vi "F11xx_FileMerger_V2.vi"() -> ()   [LabVIEW 2018]
uses:
  <vilib>/Utility/file.llb/Read From Spreadsheet File (string).vi
  <vilib>/Utility/file.llb/Write To Spreadsheet File (string).vi
panel:
  in  "Header Row":i32=42
  out "Array 4":i32[](array[numeric])=[37, 36, 36, 36, 36, 36, 36, 36, 36, 36, 36, 36, 36, 36, 36, 36, 36, 36, 36, 36, 36, 36]
  out "Array 3":bool[](array[boolean])
  out "Array 2":string[](array[string])=["10", "11", "12", "13", "14", "15", "16", "17", "18", "19", "1", "20", "21", "22", "2", "3", "4", "5", "6", "7", "8", "9"]
  out "Boolean":bool
  in  "Write to File":bool
  in  "Folder":path=path "\\\\Corpmxl0251xct\\c/IdtATE/Results/Loadbrd _r2_firstlook_F1150_080811/EvKit Plunge"
  in  "Target File":path=path "\\\\Corpmxl0251xct\\c/IdtATE/Results/Loadbrd _r2_firstlook_F1150_080811/EvKit Plunge/Loadbrd _r2_firstlook_F1150_080811_SN_1Thru22.csv"
  in  "offset (0) 2":i32=40
  in  "offset (0)":i32=11
  out "Array":string[](array[string])=["9", "9", "9", "9", "9", "9", "9", "9", "9", "9", "9", "9", "9", "9", "9", "9", "9", "9", "9", "9", "9", "9", "9", "9", "9", "9", "9", "9", "9", "9", "9", "9", "9", "9", "9", "9"]
  out "element":i32=36
  out "filenames":string[](array[string])=["Loadbrd _r2_firstlook_F1150_080811_SN_1-10_151403.csv", "Loadbrd _r2_firstlook_F1150_080811_SN_1-11_152349.csv", "Loadbrd _r2_firstlook_F1150_080811_SN_1-12_153322.csv", "Loadbrd _r2_firstlook_F1150_080811_SN_1-13_154231.csv", "Loadbrd _r2_firstlook_F1150_080811_SN_1-14_155132.csv", "Loadbrd _r2_firstlook_F1150_080811_SN_1-15_160102.csv", "Loadbrd _r2_firstlook_F1150_080811_SN_1-16_161750.csv", "Loadbrd _r2_firstlook_F1150_080811_SN_1-17_162638.csv", "Loadbrd _r2_firstlook_F1150_080811_SN_1-18_163501.csv", "Loadbrd _r2_firstlook_F1150_080811_SN_1-19_164508.csv", "Loadbrd _r2_firstlook_F1150_080811_SN_1-1_134125.csv", "Loadbrd _r2_firstlook_F1150_080811_SN_1-20_165401.csv", "Loadbrd _r2_firstlook_F1150_080811_SN_1-21_170335.csv", "Loadbrd _r2_firstlook_F1150_080811_SN_1-22_171202.csv", "Loadbrd _r2_firstlook_F1150_080811_SN_1-2_135257.csv", "Loadbrd _r2_firstlook_F1150_080811_SN_1-3_140438.csv", "Loadbrd _r2_firstlook_F1150_080811_SN_1-4_141457.csv", "Loadbrd _r2_firstlook_F1150_080811_SN_1-5_142448.csv", "Loadbrd _r2_firstlook_F1150_080811_SN_1-6_143320.csv", "Loadbrd _r2_firstlook_F1150_080811_SN_1-7_144223.csv", "Loadbrd _r2_firstlook_F1150_080811_SN_1-8_145159.csv", "Loadbrd _r2_firstlook_F1150_080811_SN_1-9_150415.csv"]
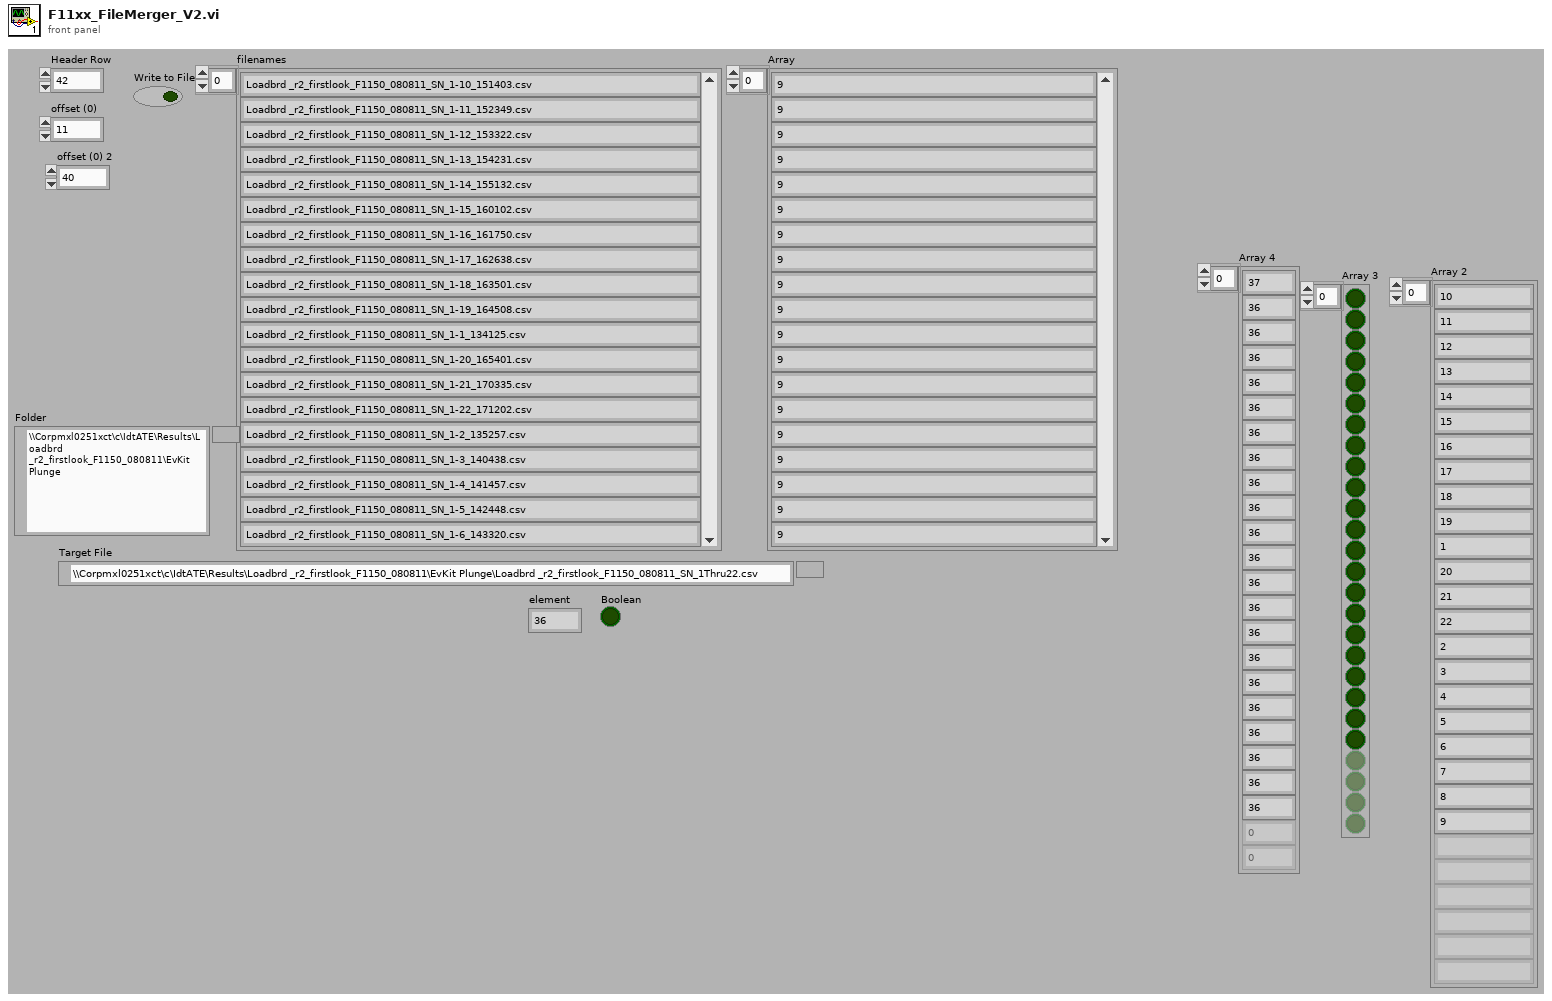
[diagram p1: front panel]
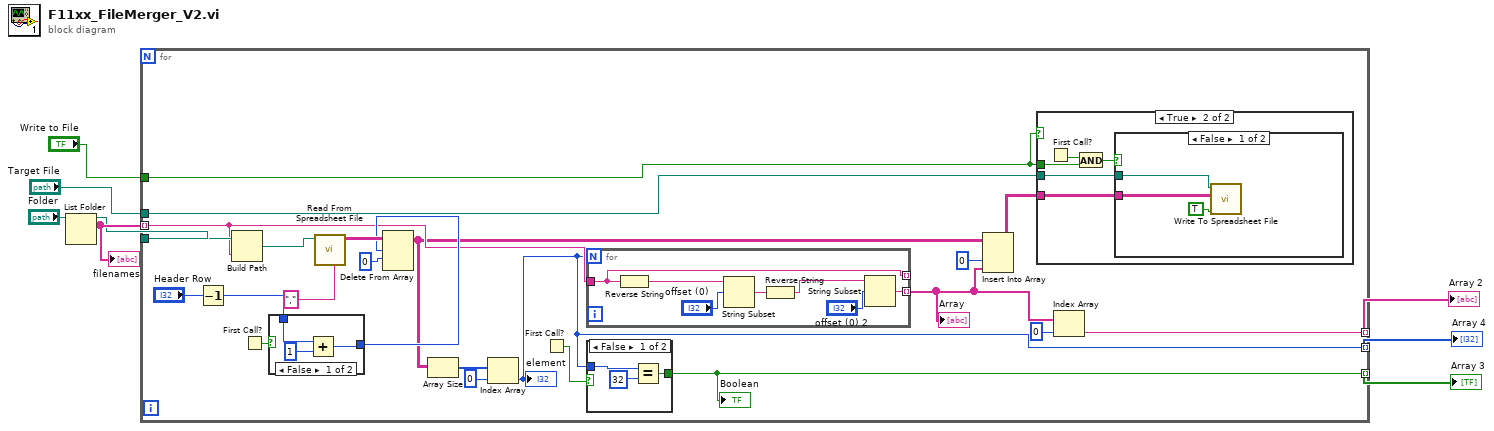
[diagram p0: block diagram]
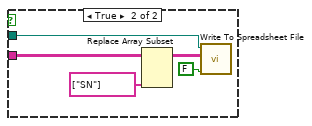
[diagram p3: hidden frame]
diagram:
  n1 = List Folder(path="Folder") -> (path out=w6:path, filenames=w7:string[])  [unwired: 3 in, 2 out]
  "filenames" <- w7
  n2 = for {
    tunnel: w7 -> [w24] mode=indexing
    tunnel: w6 -> [w28]
    tunnel: "Target File" -> [w21]
    tunnel: "Write to File" -> [w11]
    tunnel: [w14] -> w3 mode=indexing
    tunnel: [w13] -> w2 mode=indexing
    tunnel: [w12] -> w1 mode=indexing
    n3 = Decrement(x="Header Row") -> (x-1=w9:i32)
    n4 = Build Path(base path=w28, name or relative path=w24) -> (appended path=w27:path)
    n5 = First Call?() -> (First Call?: T/F=w22:bool)
    n6 = case shown="False" w22 {
      tunnel: [w49 w51] -> w30
      tunnel: w9 -> [w50 w51]
      frame False {
        n7 = Add(x=w50, y=1) -> (x+y=w49:i32)
      }
      frame True {
      }
    }
    n8 = call-poly <vilib>:"Read From Spreadsheet File.vi"("delimiter (\\t)"="," ("delimiter (\\t)"), "file path (dialog if empty)"=w27) -> ("all rows"=w31:string[][])  [unwired: 5 in, 4 out]
    n9 = Delete From Array(array=w31, length=w30, index (row)=0) -> (array with subset deleted=w23:string[][])  [unwired: 1 in, 1 out]
    n10 = Array Size(array=w23) -> (size(s)=w26:i32[])
    n11 = Index Array(array=w26, index=0) -> (element=w12:i32)
    "element" <- w12
    n12 = First Call?() -> (First Call?: T/F=w17:bool)
    n13 = for {
      N: w12 -> [_]
      tunnel: [w57] -> _ mode=indexing
      tunnel: w24 -> [w57]
      tunnel: [w53] -> w16 mode=indexing
      n14 = Reverse String(1:w57) -> (0:w56:string)
      n15 = String Subset(string=w56, offset (0)="offset (0)") -> (substring=w58:string)  [unwired: 1 in]
      n16 = Reverse String(1:w58) -> (0:w54:string)
      n17 = String Subset(string=w54, offset (0)="offset (0) 2") -> (substring=w53:string)  [unwired: 1 in]
    }
    "Array" <- w16
    n18 = case shown="False" w17 {
      tunnel: w12 -> [w47 _]
      tunnel: [w45 _] -> w13
      frame False {
        n19 = Equal?(x=w47, y=32) -> (x = y?=w45:bool)
      }
      frame True {
      }
    }
    "Boolean" <- w13
    n20 = Insert Into Array(array=w23, index (col)=0 ("disabled index (col)"), new element=w16) -> (w19:string[][])  [unwired: 1 in]
    n21 = case shown="True" w11 {
      tunnel: w21 -> [_ w36]
      tunnel: w19 -> [_ w35]
      tunnel: w11 -> [_ w32]
      frame False {
      }
      frame True {
        n22 = First Call?() -> (First Call?: T/F=w34:bool)
        n23 = And(x=w34, y=w32) -> (x .and. y?=w33:bool)
        n24 = case shown="False" w33 {
          tunnel: w35 -> [w39 w42]
          tunnel: w36 -> [w37 w43]
          frame False {
            n25 = call-poly <vilib>:"Write To Spreadsheet File.vi"("append to file? (new file:F)"=TRUE, "2D data"=w39, "file path (dialog if empty)"=w37) -> ()  [unwired: 5 in, 1 out]
          }
          frame True {
            n26 = Replace Array Subset(array=w42, new element=string[] ["SN"] ("new element/subarray")) -> (w40:string[][])  [unwired: 2 in]
            n27 = call-poly <vilib>:"Write To Spreadsheet File.vi"("append to file? (new file:F)"=FALSE, "2D data"=w40, "file path (dialog if empty)"=w43) -> ()  [unwired: 5 in, 1 out]
          }
        }
      }
    }
    n28 = Index Array(array=w16, index=0) -> (element=w14:string)
  }
  "Array 2" <- w3
  "Array 3" <- w2
  "Array 4" <- w1
